vi "GUI.vi"() -> ()   [LabVIEW 2020]
uses:
  <vilib>/DAQmx/read.llb/DAQmx Read (Analog DBL 1Chan 1Samp).vi
  <vilib>/DAQmx/miscellaneous.llb/DAQmx Fill In Error Info.vi
  <vilib>/Utility/file.llb/Write Delimited Spreadsheet (string).vi
  <vilib>/Utility/file.llb/Write Delimited Spreadsheet (DBL).vi
  <vilib>/express/express arith-compare/Formula/XNode/ExpressFormulaBlockNode.xnode
panel:
  in  "Seconds per data point (sec)":dbl
  in  "stop":bool
  in  "Tab Control":enum32{"Overview", "Graphs"}(tab)
  in  "Start Button":bool
  out "NTU":dbl
  out "NTU":dbl
  out "NTU":dbl
  out "%":dbl
  out "L/s":dbl
  out "L/s":dbl
  in  "Gauge":bool
  in  "Coagulant Dose":bool
  in  "Switch":bool
  in  "Pump 2":bool
  in  "Pump 1":bool
  in  "UV254":bool
  in  "PID 3":bool
  in  "PID 2":bool
  in  "Valve 2":bool
  in  "Flow 2":bool
  in  "NTU 2":bool
  in  "NTU 3":bool
  in  "Flow 1":bool
  in  "Valve 1":bool
  in  "PID 1":bool
  in  "NTU 1":bool
  out "L/s":cluster{dbl[], dbl[]}[](graph)
  out "NTU":cluster{dbl[], dbl[]}[](graph)
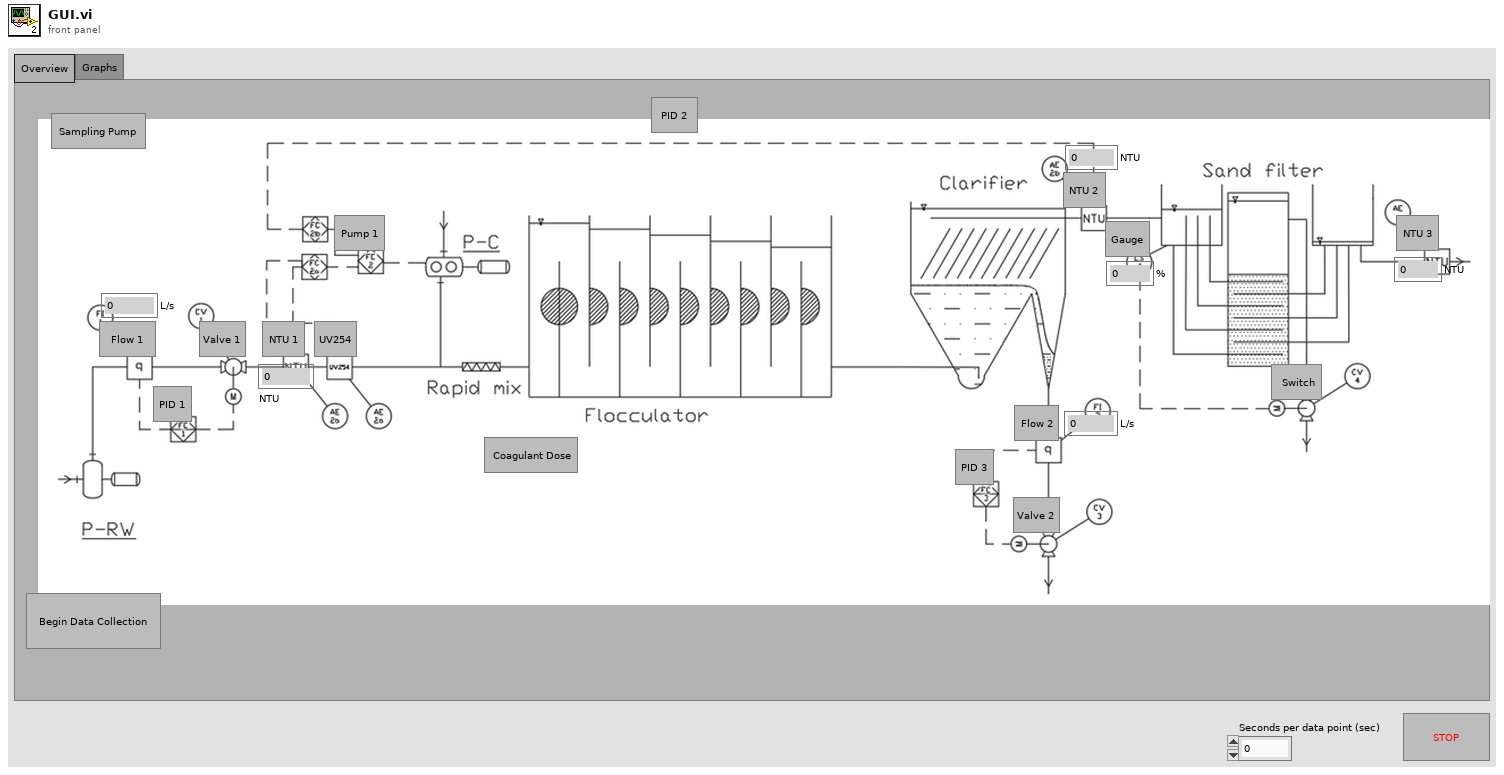
[diagram p1: front panel]
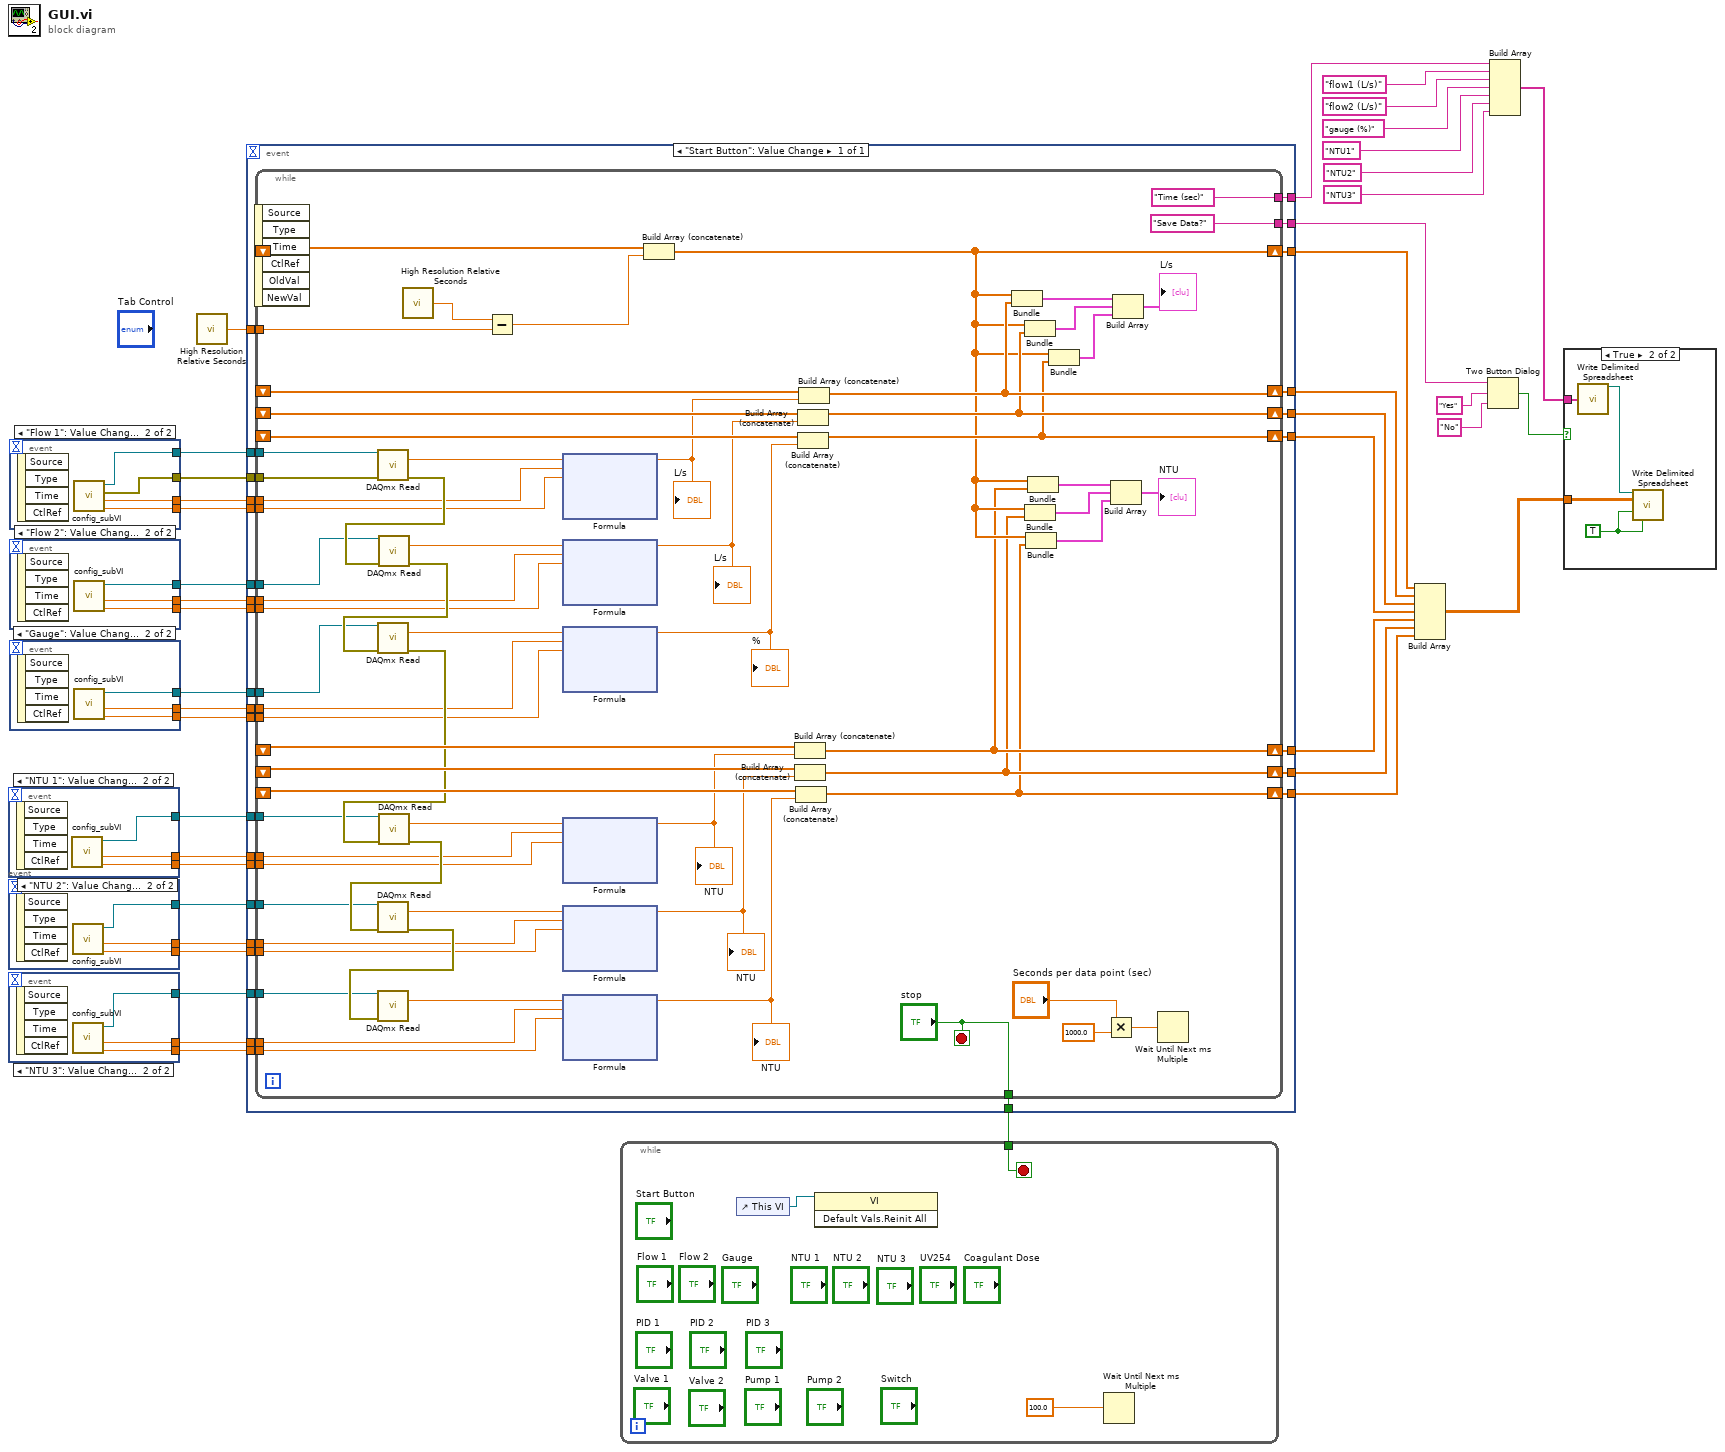
[diagram p0: block diagram]
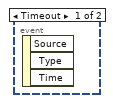
[diagram p3: hidden frame]
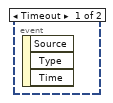
[diagram p4: hidden frame]
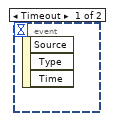
[diagram p5: hidden frame]
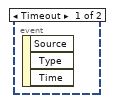
[diagram p6: hidden frame]
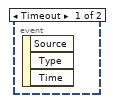
[diagram p7: hidden frame]
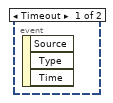
[diagram p8: hidden frame]
diagram:
  n1 = event shown="[1] \"NTU 1\": Value Change" {
    selector: _ -> [_ _]
    dyn-events: _ -> [_ _]
    timeout: _ -> [_ _]
    tunnel: [_ w44] -> w31
    tunnel: [_ w43] -> w30
    tunnel: [_ w42] -> w29
    event Timeout {
      n2 = event-data() -> ()  [unwired: 1 in, 3 out]
    }
    event "NTU 1": Value Change {
      n3 = event-data() -> ()  [unwired: 1 in, 4 out]
      n4 = call "config_subVI.vi"() -> ("B out"=w44:dbl, "A out"=w43:dbl, "task out"=w42:refnum<k21>)  [unwired: 8 in, 1 out]
    }
  }
  n5 = event shown="[1] \"NTU 2\": Value Change" {
    selector: _ -> [_ _]
    dyn-events: _ -> [_ _]
    timeout: _ -> [_ _]
    tunnel: [_ w47] -> w28
    tunnel: [_ w46] -> w27
    tunnel: [_ w45] -> w26
    event Timeout {
      n6 = event-data() -> ()  [unwired: 1 in, 3 out]
    }
    event "NTU 2": Value Change {
      n7 = event-data() -> ()  [unwired: 1 in, 4 out]
      n8 = call "config_subVI.vi"() -> ("B out"=w47:dbl, "A out"=w46:dbl, "task out"=w45:refnum<k21>)  [unwired: 8 in, 1 out]
    }
  }
  n9 = event shown="[1] \"NTU 3\": Value Change" {
    selector: _ -> [_ _]
    dyn-events: _ -> [_ _]
    timeout: _ -> [_ _]
    tunnel: [_ w50] -> w25
    tunnel: [_ w49] -> w24
    tunnel: [_ w48] -> w2
    event Timeout {
      n10 = event-data() -> ()  [unwired: 1 in, 3 out]
    }
    event "NTU 3": Value Change {
      n11 = event-data() -> ()  [unwired: 1 in, 4 out]
      n12 = call "config_subVI.vi"() -> ("B out"=w50:dbl, "A out"=w49:dbl, "task out"=w48:refnum<k21>)  [unwired: 8 in, 1 out]
    }
  }
  n13 = event shown="[1] \"Flow 1\": Value Change" {
    selector: _ -> [_ _]
    dyn-events: _ -> [_ _]
    timeout: _ -> [_ _]
    tunnel: [_ w54] -> w41
    tunnel: [_ w53] -> w40
    tunnel: [_ w52] -> w39
    tunnel: [_ w51] -> w38
    event Timeout {
      n14 = event-data() -> ()  [unwired: 1 in, 3 out]
    }
    event "Flow 1": Value Change {
      n15 = event-data() -> ()  [unwired: 1 in, 4 out]
      n16 = call "config_subVI.vi"() -> ("B out"=w54:dbl, "A out"=w53:dbl, "error out"=w52:errorcluster, "task out"=w51:refnum<k21>)  [unwired: 8 in]
    }
  }
  n17 = event shown="[1] \"Flow 2\": Value Change" {
    selector: _ -> [_ _]
    dyn-events: _ -> [_ _]
    timeout: _ -> [_ _]
    tunnel: [_ w57] -> w37
    tunnel: [_ w56] -> w36
    tunnel: [_ w55] -> w35
    event Timeout {
      n18 = event-data() -> ()  [unwired: 1 in, 3 out]
    }
    event "Flow 2": Value Change {
      n19 = event-data() -> ()  [unwired: 1 in, 4 out]
      n20 = call "config_subVI.vi"() -> ("B out"=w57:dbl, "A out"=w56:dbl, "task out"=w55:refnum<k21>)  [unwired: 8 in, 1 out]
    }
  }
  n21 = event shown="[1] \"Gauge\": Value Change" {
    selector: _ -> [_ _]
    dyn-events: _ -> [_ _]
    timeout: _ -> [_ _]
    tunnel: [_ w60] -> w34
    tunnel: [_ w59] -> w33
    tunnel: [_ w58] -> w32
    event Timeout {
      n22 = event-data() -> ()  [unwired: 1 in, 3 out]
    }
    event "Gauge": Value Change {
      n23 = event-data() -> ()  [unwired: 1 in, 4 out]
      n24 = call "config_subVI.vi"() -> ("B out"=w60:dbl, "A out"=w59:dbl, "task out"=w58:refnum<k21>)  [unwired: 8 in, 1 out]
    }
  }
  n25 = call <vilib>:"High Resolution Relative Seconds.vi"() -> ("relative seconds"=w3:dbl)
  n26 = event shown="[0] \"Start Button\": Value Change" {
    selector: _ -> [_]
    dyn-events: _ -> [_]
    timeout: _ -> [_]
    tunnel: w41 -> [w90]
    tunnel: w40 -> [w89]
    tunnel: w39 -> [w88]
    tunnel: w38 -> [w87]
    tunnel: w37 -> [w86]
    tunnel: w36 -> [w85]
    tunnel: w35 -> [w84]
    tunnel: w34 -> [w83]
    tunnel: w33 -> [w82]
    tunnel: w32 -> [w81]
    tunnel: w31 -> [w80]
    tunnel: w30 -> [w79]
    tunnel: w29 -> [w78]
    tunnel: w28 -> [w77]
    tunnel: w27 -> [w76]
    tunnel: w26 -> [w75]
    tunnel: w25 -> [w74]
    tunnel: w24 -> [w73]
    tunnel: [w72] -> w23
    tunnel: [w71] -> w22
    tunnel: [w70] -> w21
    tunnel: [w69] -> w20
    tunnel: [w68] -> w19
    tunnel: [w67] -> w18
    tunnel: [w66] -> w17
    tunnel: [w65] -> w16
    tunnel: [w64] -> w9
    tunnel: w3 -> [w63]
    tunnel: w2 -> [w62]
    tunnel: [w61] -> w1
    event "Start Button": Value Change {
      n27 = event-data() -> ()  [unwired: 1 in, 6 out]
      n28 = while {
        shift-right: [w135] -> w72
        shift-left: _ -> [w155]
        shift-right: [w153] -> w71
        shift-left: _ -> [w154]
        shift-right: [w147] -> w70
        shift-left: _ -> [w148]
        shift-right: [w140] -> w69
        shift-left: _ -> [w141]
        shift-right: [w127] -> w66
        shift-left: _ -> [w130]
        shift-right: [w126] -> w67
        shift-left: _ -> [w129]
        shift-right: [w125] -> w68
        shift-left: _ -> [w128]
        tunnel: w90 -> [w113]
        tunnel: w89 -> [w112]
        tunnel: w88 -> [w111]
        tunnel: w87 -> [w110]
        tunnel: w86 -> [w109]
        tunnel: w85 -> [w108]
        tunnel: w84 -> [w107]
        tunnel: w83 -> [w106]
        tunnel: w82 -> [w105]
        tunnel: w81 -> [w104]
        tunnel: w80 -> [w103]
        tunnel: w79 -> [w102]
        tunnel: w78 -> [w101]
        tunnel: w77 -> [w100]
        tunnel: w76 -> [w99]
        tunnel: w75 -> [w98]
        tunnel: w74 -> [w92]
        tunnel: w73 -> [w97]
        tunnel: w62 -> [w96]
        tunnel: ["Time (sec)"] -> w65
        tunnel: ["Save Data?" ("message")] -> w64
        tunnel: w63 -> [w93]
        tunnel: ["stop"] -> w61
        stop <- "stop" stop-if-true
        n29 = call-poly <vilib>:"DAQmx Read.vi"("task/channels in"=w110, "error in"=w111) -> ("data"=w138:dbl, "error out"=w118:errorcluster)  [unwired: 11 in, 1 out]
        n30 = call-poly <vilib>:"DAQmx Read.vi"("task/channels in"=w107, "error in"=w118) -> ("data"=w137:dbl, "error out"=w117:errorcluster)  [unwired: 11 in, 1 out]
        n31 = call-poly <vilib>:"DAQmx Read.vi"("task/channels in"=w104, "error in"=w117) -> ("data"=w136:dbl, "error out"=w116:errorcluster)  [unwired: 11 in, 1 out]
        n32 = call-poly <vilib>:"DAQmx Read.vi"("task/channels in"=w101, "error in"=w116) -> ("data"=w133:dbl, "error out"=w115:errorcluster)  [unwired: 11 in, 1 out]
        n33 = call-poly <vilib>:"DAQmx Read.vi"("task/channels in"=w98, "error in"=w115) -> ("data"=w132:dbl, "error out"=w114:errorcluster)  [unwired: 11 in, 1 out]
        n34 = call-poly <vilib>:"DAQmx Read.vi"("task/channels in"=w96, "error in"=w114) -> ("data"=w131:dbl)  [unwired: 11 in, 2 out]
        n35 = call <vilib>:"High Resolution Relative Seconds.vi"() -> ("relative seconds"=w157:dbl)
        n36 = Subtract(x=w157, y=w93) -> (x-y=w156:dbl)
        n37 = xnode "Formula"("data"=w138, "A"=w112, "B"=w113) -> ("Result"=w124:dbl)  [unwired: 1 in, 1 out]
        "L/s" <- w124
        n38 = xnode "Formula"("data"=w137, "A"=w108, "B"=w109) -> ("Result"=w123:dbl)  [unwired: 1 in, 1 out]
        "L/s" <- w123
        n39 = xnode "Formula"("data"=w136, "A"=w105, "B"=w106) -> ("Result"=w122:dbl)  [unwired: 1 in, 1 out]
        "%" <- w122
        n40 = xnode "Formula"("data"=w133, "A"=w102, "B"=w103) -> ("Result"=w119:dbl)  [unwired: 1 in, 1 out]
        "NTU" <- w119
        n41 = xnode "Formula"("data"=w132, "A"=w99, "B"=w100) -> ("Result"=w120:dbl)  [unwired: 1 in, 1 out]
        "NTU" <- w120
        n42 = xnode "Formula"("data"=w131, "A"=w97, "B"=w92) -> ("Result"=w121:dbl)  [unwired: 1 in, 1 out]
        "NTU" <- w121
        n43 = Build Array (concatenate)(w155, w156) -> (w135:dbl[])
        n44 = Build Array (concatenate)(w130, w119) -> (w127:dbl[])
        n45 = Build Array (concatenate)(w129, w120) -> (w126:dbl[])
        n46 = Build Array (concatenate)(w128, w121) -> (w125:dbl[])
        n47 = Build Array (concatenate)(w148, w123) -> (w147:dbl[])
        n48 = Build Array (concatenate)(w141, w122) -> (w140:dbl[])
        n49 = Build Array (concatenate)(w154, w124) -> (w153:dbl[])
        n50 = Bundle(w135, w153) -> (w152:cluster{dbl[], dbl[]})  [unwired: 1 in]
        n51 = Bundle(w135, w147) -> (w145:cluster{dbl[], dbl[]})  [unwired: 1 in]
        n52 = Bundle(w135, w126) -> (w142:cluster{dbl[], dbl[]})  [unwired: 1 in]
        n53 = Bundle(w135, w125) -> (w134:cluster{dbl[], dbl[]})  [unwired: 1 in]
        n54 = Bundle(w135, w127) -> (w143:cluster{dbl[], dbl[]})  [unwired: 1 in]
        n55 = Bundle(w135, w140) -> (w139:cluster{dbl[], dbl[]})  [unwired: 1 in]
        n56 = Multiply(x="Seconds per data point (sec)", y=1000.0) -> (x*y=w150:dbl)
        n57 = Build Array(w143, w142, w134) -> (→"NTU":cluster{dbl[], dbl[]}[])
        n58 = Build Array(w152, w145, w139) -> (→"L/s":cluster{dbl[], dbl[]}[])
        n59 = Wait Until Next ms Multiple(millisecond multiple=w150) -> ()  [unwired: 1 out]
      }
    }
  }
  n60 = while {
    tunnel: w1 -> [w230]
    stop <- w230 stop-if-true
    n61 = control-ref of="This VI"() -> (w232:refnum<vi>)
    n62 = invoke class="VI" method="Default Vals.Reinit All"(reference=w232) -> ()  [unwired: 2 in, 3 out]
    n63 = Wait Until Next ms Multiple(millisecond multiple=100.0 ("y")) -> ()  [unwired: 1 out]
  }
  n64 = Build Array(w23, w22, w21, w20, w17, w18, w19) -> (w4:dbl[][])
  n65 = Two Button Dialog(message=w9, 1:"No" ("F button name (\"Cancel\")"), 2:"Yes" ("T button name (\"OK\")")) -> (T button?=w5:bool)
  n66 = Build Array(w16, "flow1 (L/s)", "flow2 (L/s)", "gauge (%)", "NTU1", "NTU2", "NTU3") -> (w6:string[])
  n67 = case shown="True" w5 {
    tunnel: w4 -> [_ w236]
    tunnel: w6 -> [_ w235]
    frame False {
    }
    frame True {
      w233 = TRUE ("transpose? (no:F)")
      n68 = call-poly <vilib>:"Write Delimited Spreadsheet.vi"("1D data"=w235) -> ("new file path (Not A Path if cancelled)"=w234:path)  [unwired: 13 in, 1 out]
      n69 = call-poly <vilib>:"Write Delimited Spreadsheet.vi"("file path (dialog if empty)"=w234, "2D data"=w236, "append to file? (new file:F)"=w233, "transpose? (no:F)"=w233) -> ()  [unwired: 10 in, 2 out]
    }
  }
